vi "Send.vi"(10 "Error":errorcluster) -> (3 "Error Msg Strategy out":refnum<class "Error Msg.lvclass">)   [LabVIEW 2021, in "Error.lvlib" / "Error Msg.lvclass"]
uses:
  Error Msg.lvclass
  Error Msg.lvclass/Error Msg.ctl
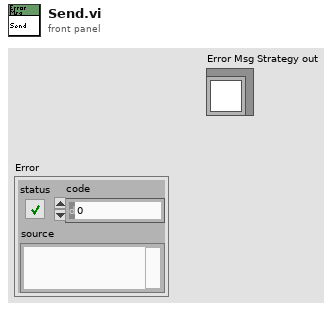
[diagram p1: front panel]
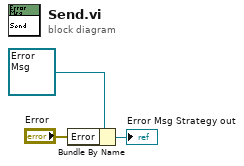
[diagram p0: block diagram]
diagram:
  n1 = Bundle By Name(cluster=refnum<class "Error Msg.lvclass"> refnum ("Error Msg Strategy out"), "Error"="Error") -> (→"Error Msg Strategy out":refnum<class "Error Msg.lvclass">)
